vi "Parse Port (Rx-UDP-SAP).vi"(8 "error in":errorcluster, 11 "node in":refnum<k20>) -> (0 "error out":errorcluster, 3 "rx udp sap port out":T1={"PayloadID"="", "UdpDstPort"=1, "UdpNumBufMessages"=0, "UdpMaxMessageSize"=128, "Parameters"=[]} {"Parameters"."Parameter"."encoding" items=["BNR", "BCD", "Discrete"]})   [LabVIEW 2020, in "AIM ARINC 664 Import.lvlib"]
uses:
  AIM ARINC 664 Import.lvlib
  _typedefs/port_rx_udp_sap.ctl
  _typedefs/frame_parameter.ctl
  _typedefs/frame_parameter_definition.ctl
  Shared/Encoding (Arinc664).ctl
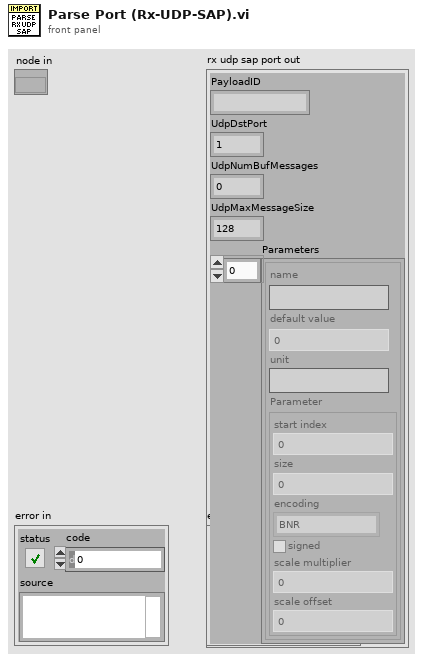
[diagram p1: front panel]
types:
  T1 = typedef "AIM ARINC 664 Import.lvlib/port_rx_udp_sap.ctl" = cluster{"PayloadID":string, "UdpDstPort":u16, "UdpNumBufMessages":u32, "UdpMaxMessageSize":u32, "Parameters":T2[]}
  T2 = typedef "AIM ARINC 664 Import.lvlib/frame_parameter.ctl" = cluster{"name":string, "default value":dbl, "unit":string, "Parameter":T3}
  T3 = typedef "AIM ARINC 664 Import.lvlib/frame_parameter_definition.ctl" = cluster{"start index":i32, "size":i32, "encoding":T4, "signed":bool, "scale multiplier":dbl, "scale offset":dbl}
  T4 = typedef "Encoding (Arinc664).ctl" = u16
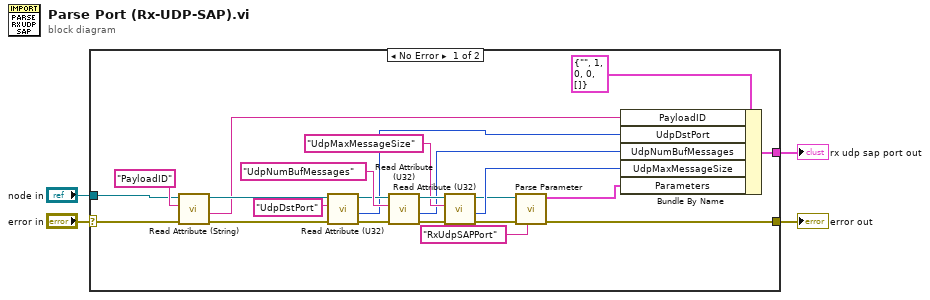
[diagram p0: block diagram]
diagram:
  n1 = case shown="No Error" "error in" {
    selector: "error in" -> [w8 w28]
    tunnel: "node in" -> [w9 _]
    tunnel: [w13 w28] -> w3
    tunnel: [w27 _] -> w1
    frame No Error {
      n2 = call "Read Attribute (String).vi"("error in"=w8, "Attribute Name"="PayloadID" ("Name"), "node in"=w9) -> ("error out"=w6:errorcluster, "value"=w5:string, "node out"=w7:refnum<k20>)  [unwired: 6 in]
      n3 = call "Read Attribute (U32).vi"("error in"=w6, "Attribute Name"="UdpDstPort" ("Tag Name"), "node in"=w7) -> ("error out"=w22:errorcluster, "value"=w16:u32, "node out"=w21:refnum<k20>)  [unwired: 6 in]
      n4 = call "Read Attribute (U32).vi"("error in"=w22, "Attribute Name"="UdpNumBufMessages" ("Tag Name"), "node in"=w21) -> ("error out"=w26:errorcluster, "value"=w18:u32, "node out"=w25:refnum<k20>)  [unwired: 6 in]
      n5 = call "Read Attribute (U32).vi"("error in"=w26, "Attribute Name"="UdpMaxMessageSize" ("Tag Name"), "node in"=w25) -> ("error out"=w14:errorcluster, "value"=w17:u32, "node out"=w15:refnum<k20>)  [unwired: 6 in]
      n6 = call "Parse Parameter.vi"("error text in"="RxUdpSAPPort", "error in"=w14, "node in"=w15) -> ("error out"=w13:errorcluster, "parametesrs"=w12:T2[])  [unwired: 7 in]
      n7 = Bundle By Name(cluster=T1 {"PayloadID"="", "UdpDstPort"=1, "UdpNumBufMessages"=0, "UdpMaxMessageSize"=0, "Parameters"=[]} ("port_tx_udp_comm"), "PayloadID"=w5, "UdpDstPort"=w16, "UdpNumBufMessages"=w18, "UdpMaxMessageSize"=w17, "Parameters"=w12) -> (w27:T1)
    }
    frame Error {
    }
  }
  "error out" <- w3
  "rx udp sap port out" <- w1
